vi "Control Path.vi"(11 "2WayValveEditorPanel in":refnum<class "2WayValveEditorPanel.lvclass">) -> (2 "Control Paths":path[](array[path]))   [LabVIEW 2020, in "VolatusGUIControls.lvlib" / "2WayValveEditorPanel.lvclass"]
uses:
  2WayValveEditorPanel.lvclass
  2WayValveEditorPanel.lvclass/2WayValveEditorPanel.ctl
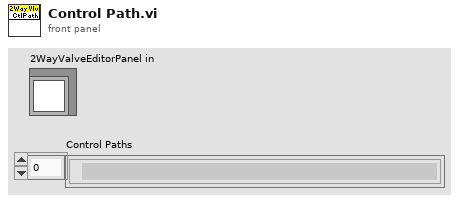
[diagram p1: front panel]
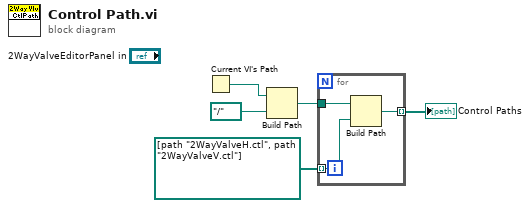
[diagram p0: block diagram]
diagram:
  n1 = Current VI's Path() -> (path=w5:path)
  n2 = Build Path(base path=w5, name or relative path=path "../..") -> (appended path=w2:path)
  n3 = for {
    tunnel: path[] [path "2WayValveH.ctl", path "2WayValveV.ctl"] -> [w7] mode=indexing
    tunnel: w2 -> [w8]
    tunnel: [w6] -> w1 mode=indexing
    n4 = Build Path(base path=w8, name or relative path=w7) -> (appended path=w6:path)
  }
  "Control Paths" <- w1
